vi "svx_DAQ_CheckXControlSize.vi"(7 "Task Configuration Pane":refnum<vi>, 8 "XControl Boolean Size Number":u32, 9 "XControl Ref":refnum<vi>) -> (0 "error out":errorcluster, 1 "Task Configuration Pane Height":u32, 2 "Update Size?":bool, 3 "XControl Ref Out":refnum<vi>)   [LabVIEW 2017, in "SVX NI-DAQmx AI Configuration XControl.xctl"]
uses:
  <vilib>/addons/Sound and Vibration/svt_DAQmx/Configuration XControl/SVX NI-DAQmx AI Configuration XControl.xctl
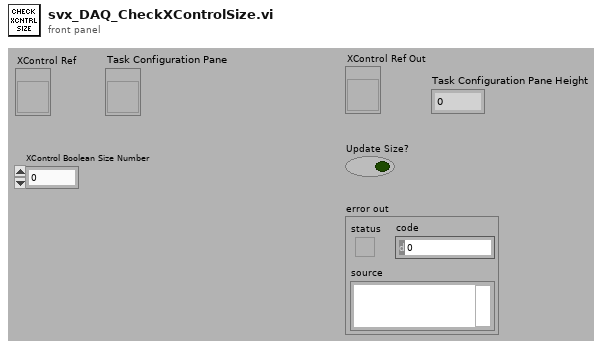
[diagram p1: front panel]
types:
  T1 = typedef "LVBoundsTypeDef.ctl" = cluster{"Width":u32, "Height":u32}
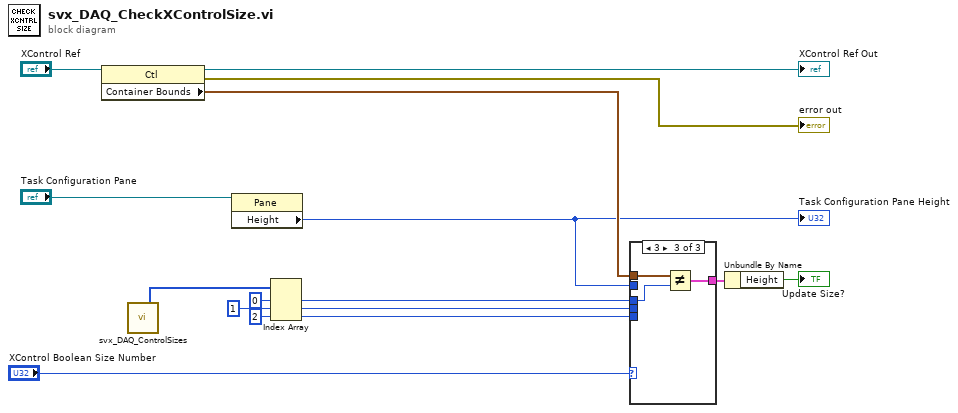
[diagram p0: block diagram]
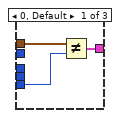
[diagram p2: hidden frame]
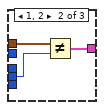
[diagram p3: hidden frame]
diagram:
  n1 = property class="Ctl"(reference="XControl Ref") -> (reference out=→"XControl Ref Out":refnum<vi>, error out=→"error out":errorcluster, "Container Bounds"=w15:T1)  [unwired: 1 in]
  n2 = call <vilib>:"svx_DAQ_ControlSizes.vi"() -> ("Task Configuration Pane Heights"=w1:u32[])  [unwired: 10 in, 5 out]
  n3 = property class="Pane"(reference="Task Configuration Pane") -> ("Height"=w2:u32)  [unwired: 1 in, 2 out]
  "Task Configuration Pane Height" <- w2
  n4 = Index Array(array=w1, index #1=0 ("index"), index #2=1 ("index"), index #3=2 ("index")) -> (element #1=w11:u32, element #2=w10:u32, element #3=w9:u32)
  n5 = case shown="3" "XControl Boolean Size Number" {
    tunnel: w15 -> [w19 w22 w25]
    tunnel: w11 -> [_ _ w24]
    tunnel: w10 -> [_ w21 _]
    tunnel: w9 -> [w18 _ _]
    tunnel: [w17 w20 w23] -> w8
    tunnel: w2 -> [_ _ _]
    frame 0, Default {
      n6 = Not Equal?(x=w19, y=w18) -> (x != y?=w17:cluster{"Width":bool, "Height":bool})
    }
    frame 1, 2 {
      n7 = Not Equal?(x=w22, y=w21) -> (x != y?=w20:cluster{"Width":bool, "Height":bool})
    }
    frame 3 {
      n8 = Not Equal?(x=w25, y=w24) -> (x != y?=w23:cluster{"Width":bool, "Height":bool})
    }
  }
  n9 = Unbundle By Name(w8) -> ("Height"=→"Update Size?":bool)
